vi "decodeMessage.vi"(8 "error in (no error)":errorcluster, 10 "MessageString":string, 11 "CameraNetworkServer in":refnum<class "CameraNetworkServer.lvclass">) -> (0 "error out":errorcluster, 2 "close":bool, 3 "CameraNetworkServer out":refnum<class "CameraNetworkServer.lvclass">)   [LabVIEW 2009, in "Hardware.lvlib" / "HWControllers.lvlib" / "CameraNetworkServer.lvclass"]
uses:
  CameraNetworkServer.lvclass
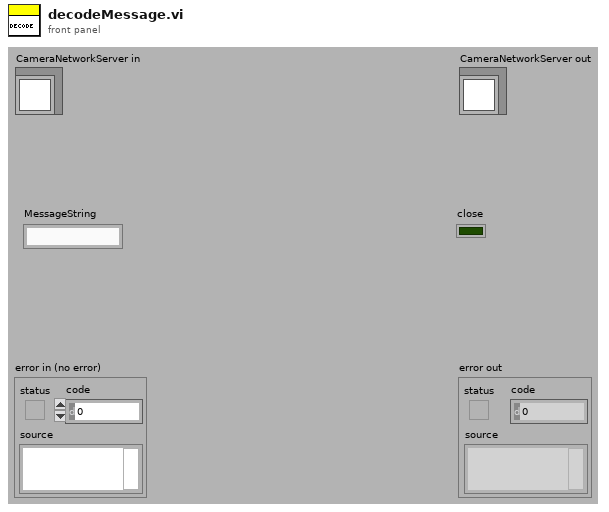
[diagram p1: front panel]
types:
  T1 = enum16{"Idle", "initialise", "configureAcquisition", "setTemperature", "getTemperature", "start", "stop", "sendImage", "close", "error", "ExitApp", "getAcquisitionStatus"}
  T2 = cluster{"Message":enum16{"Idle", "initialise", "configureAcquisition", "setTemperature", "getTemperature", "start", "stop", "sendImage", "close", "error", "ExitApp", "getAcquisitionStatus"}, "Data":variant}
  T3 = enum16{"Idle", "initialise", "configureAcquisition", "setTemperature", "getTemperature", "start", "stop", "sendImage", "close", "error", "ExitApp"}
  T4 = cluster{"Message":enum16{"Idle", "initialise", "configureAcquisition", "setTemperature", "getTemperature", "start", "stop", "sendImage", "close", "error", "ExitApp", "getAcquisitionStatus"}, "Data":variant}[]
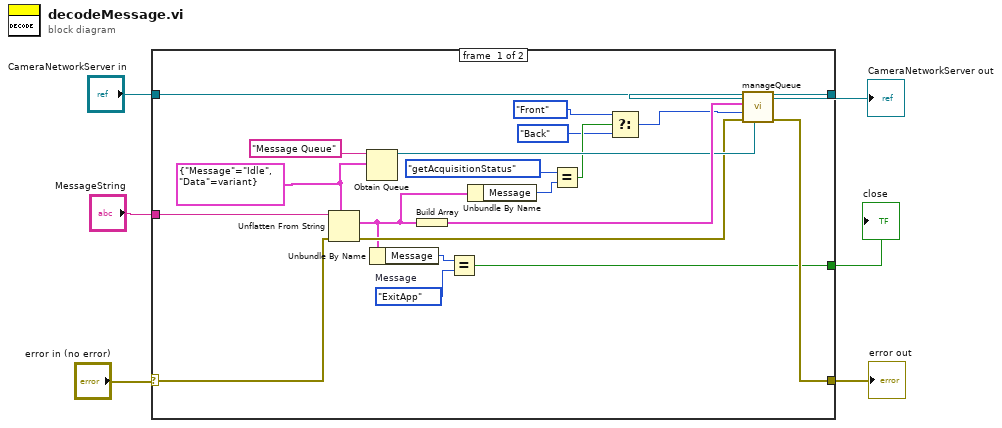
[diagram p0: block diagram]
diagram:
  n1 = case shown="No Error" "error in (no error)" {
    selector: "error in (no error)" -> [w16 w27]
    tunnel: [w24 w28] -> w6
    tunnel: "CameraNetworkServer in" -> [w25 w28]
    tunnel: [w22 w27] -> w3
    tunnel: "MessageString" -> [w26 _]
    tunnel: [w17 _] -> w1
    frame #0 {
      w14 = T2 {"Message"=enum."Idle", "Data"=variant}
      w18 = T3."ExitApp"  # Message
      n2 = Unflatten From String(type=w14, binary string=w26, error in (no error)=w16) -> (value=w13:T2, error out=w15:errorcluster)  [unwired: 2 in, 1 out]
      n3 = Obtain Queue(name (unnamed)="Message Queue", element data type=w14) -> (queue out=w21:refnum<queue>)  [unwired: 3 in, 2 out]
      n4 = Unbundle By Name(w13) -> ("Message"=w19:T1)
      n5 = Build Array(w13) -> (w23:T4)
      n6 = Equal?(x=w19, y=w18) -> (x = y?=w17:bool)
      n7 = Unbundle By Name(w13) -> ("Message"=w12:T1)
      n8 = Equal?(x=T1."getAcquisitionStatus" ("Message"), y=w12) -> (x = y?=w10:bool)
      n9 = Select(t=enum16{"Back", "Front", "Replace"}."Front" ("FNs"), s=w10, f=enum16{"Back", "Front", "Replace"}."Back" ("FNs")) -> (s? t:f=w7:enum16{"Back", "Front", "Replace"})
      n10 = call "manageQueue.vi"("MessageQRef"=w21, "error in (no error)"=w15, "FNs"=w7, "Message"=w23, "CameraNetworkClient in"=w25) -> ("error out"=w22:errorcluster, "CameraNetworkClient out"=w24:refnum<class "CameraNetworkServer.lvclass">)  [unwired: 5 in]
    }
    frame #1 {
    }
  }
  "error out" <- w3
  "CameraNetworkServer out" <- w6
  "close" <- w1
